vi "PADMINI_AUTO_BARCODE_STATUS4.vi"(7 "Enum":enum16{"Read", "Write"}(ring), 8 "error in (no error)":errorcluster, 10 "I/P":u16) -> (0 "error out":errorcluster, 2 "O/P":u16)   [LabVIEW 2017]
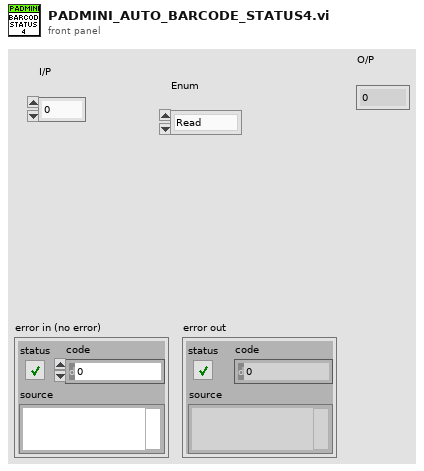
[diagram p1: front panel]
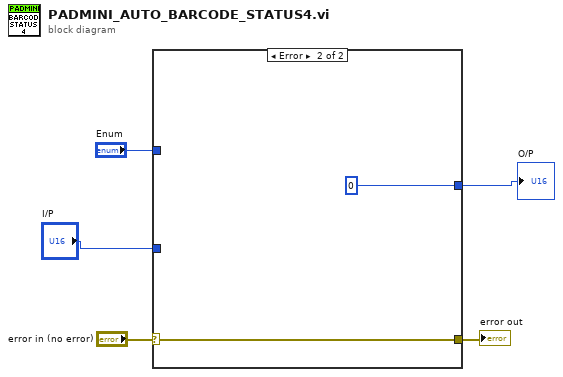
[diagram p0: block diagram]
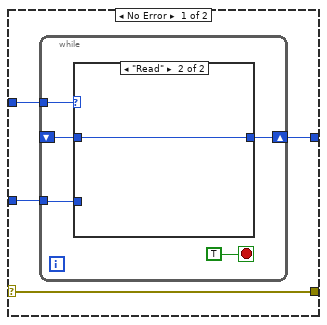
[diagram p2: hidden frame]
diagram:
  n1 = case shown="Error" "error in (no error)" {
    selector: "error in (no error)" -> [w6 w18]
    tunnel: "Enum" -> [w9 _]
    tunnel: "I/P" -> [w8 _]
    tunnel: [w7 u16 0] -> w1
    tunnel: [w6 w18] -> w3
    frame No Error {
      n2 = while {
        tunnel: w9 -> [w14]
        shift-right: [w12] -> w7
        shift-left: _ -> [w11]
        tunnel: w8 -> [w13]
        stop <- TRUE stop-if-true
        n3 = case shown="\"Read\"" w14 {
          tunnel: [w15 w16] -> w12
          tunnel: w13 -> [w15 _]
          tunnel: w11 -> [_ w16]
          frame "Write", Default {
          }
          frame "Read" {
          }
        }
      }
    }
    frame Error {
    }
  }
  "error out" <- w3
  "O/P" <- w1
